vi "Write Server address.vi"(8 "error in (no error)":errorcluster, 10 "Server address":string="192.168.1.100", 11 "Red Pitaya Digitizer in":refnum<class "Red Pitaya Digitizer.lvclass">) -> (0 "error out":errorcluster, 3 "Red Pitaya Digitizer out":refnum<class "Red Pitaya Digitizer.lvclass">)   [LabVIEW 2018, in "Red Pitaya Digitizer.lvclass"]
uses:
  Red Pitaya Digitizer.lvclass
  Red Pitaya Digitizer.lvclass/Red Pitaya Digitizer.ctl
  RP Core/RP Instrument/RP Instrument.lvclass
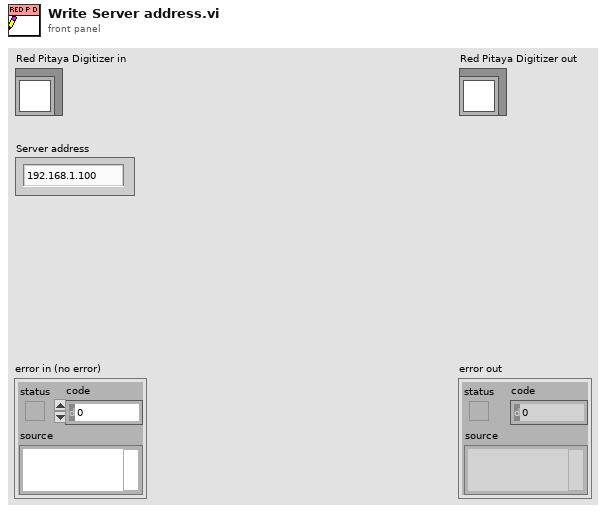
[diagram p1: front panel]
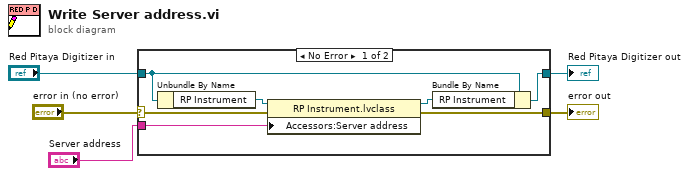
[diagram p0: block diagram]
diagram:
  n1 = case shown="No Error" "error in (no error)" {
    selector: "error in (no error)" -> [w7 w13]
    tunnel: [w6 w13] -> w4
    tunnel: [w12 w14] -> w2
    tunnel: "Red Pitaya Digitizer in" -> [w9 w14]
    tunnel: "Server address" -> [w10 _]
    frame No Error {
      n2 = Unbundle By Name(w9) -> ("RP Instrument"=w11:refnum<class "RP Instrument.lvclass">)
      n3 = property class="RP Instrument.lvclass"(reference=w11, error in=w7, "Accessors:Server address"=w10) -> (reference out=w8:refnum<class "RP Instrument.lvclass">, error out=w6:errorcluster)
      n4 = Bundle By Name(cluster=w9, "RP Instrument"=w8) -> (w12:refnum<class "Red Pitaya Digitizer.lvclass">)
    }
    frame Error {
    }
  }
  "error out" <- w4
  "Red Pitaya Digitizer out" <- w2
